vi "OP600ZP_SCANequipements.vi"(8 "Errin":errorcluster caption="errin", 10 "Chaîne":string="Log et conf\\Config.ini", 11 "pathin":path=path "D:/CODE/02 SLIM ZEN") -> (0 "errout":errorcluster={"status"=TRUE, "code"=0, "source"="PCAN_CHANNEL ILLEGAL"}, 1 "KO?":bool=TRUE, 2 "ST5520":refnum<visa-resource-name>, 3 "VISA OUT":T1, 4 "BT3564":refnum<visa-resource-name>, 6 "ALIM":refnum<visa-resource-name>)   [LabVIEW 2020]
doc: "Ce vi il détecte la presence des équipements"
uses:
  VG/VG_BT3564.vi
  VG/VG_ALIM.vi
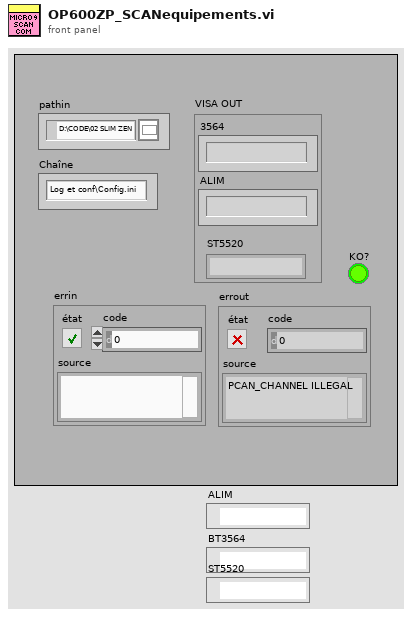
[diagram p1: front panel]
types:
  T1 = cluster{"3564":string, "ALIM":string, "ST5520":string}
  T2 = cluster{"3564":string, "ST5520":string, "ALIM":string}
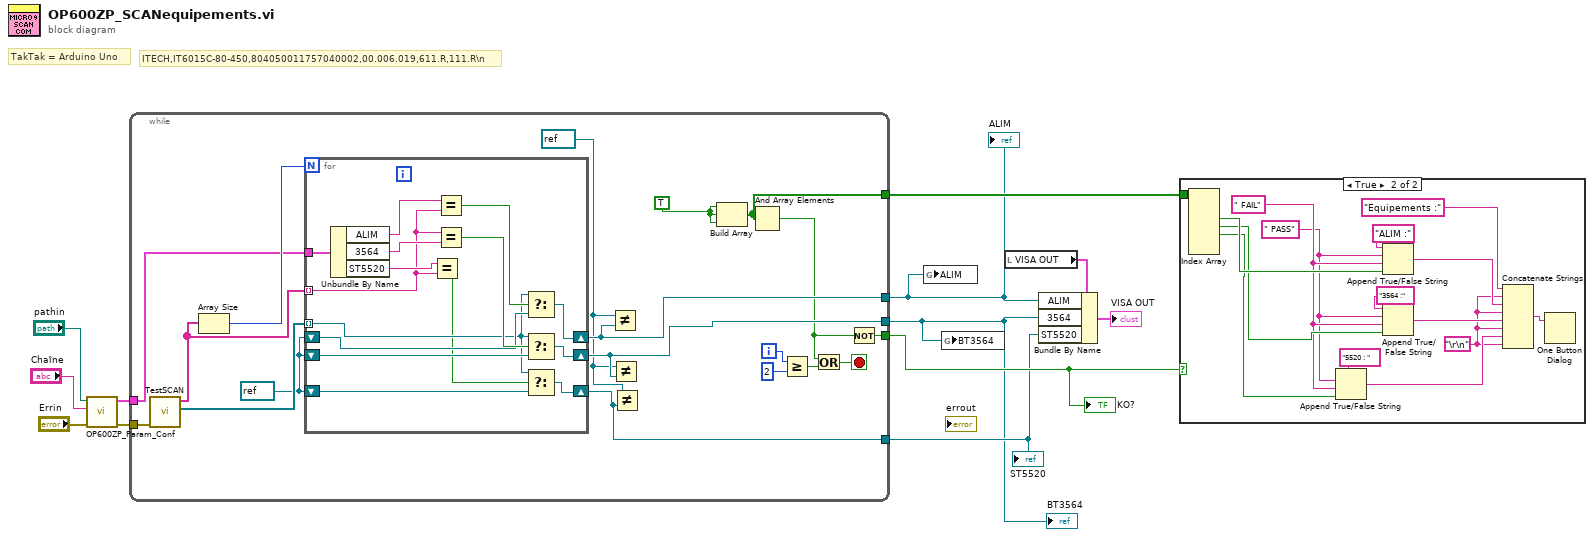
[diagram p0: block diagram]
diagram:
  # "TakTak = Arduino Uno"
  # "ITECH,IT6015C-80-450,804050011757040002,00.006.019,611.R,111.R\\n"
  n1 = call "OP600ZP_Param_Conf.vi"("errin"="Errin", "Chaîne"="Chaîne", "pathin"="pathin") -> ("errout"=w9:errorcluster, "VISA OUT"=w8:T2)  [unwired: 7 in]
  n2 = while {
    tunnel: [w20] -> w2
    tunnel: [w19] -> w1
    tunnel: w9 -> [w29]
    tunnel: [w24] -> w12
    tunnel: w8 -> [w21]
    tunnel: [w17] -> w11
    tunnel: [w14] -> w3
    i -> [w23]
    stop <- w26 stop-if-true
    w13 = TRUE ("élément")
    w15 = refnum<visa-resource-name> refnum ("x")
    w16 = refnum<visa-resource-name> refnum ("VISA resource name out")
    n3 = call <userlib>:"TestSCAN.vi"("errin"=w29) -> ("Tableau 2"=w27:refnum<visa-resource-name>[], "Tableau"=w28:string[])  [unwired: 8 in, 1 out]
    n4 = Array Size(array=w28) -> (size(s)=w30:i32)
    n5 = for {
      N: w30 -> [_]
      shift-right: [w43] -> w20
      shift-left: w16 -> [w41]
      shift-right: [w42] -> w19
      shift-left: w16 -> [w40]
      tunnel: w28 -> [w32] mode=indexing
      tunnel: w21 -> [w39]
      shift-right: [w35] -> w14
      shift-left: w16 -> [w36]
      tunnel: w27 -> [w34] mode=indexing
      n6 = Unbundle By Name(w39) -> ("ALIM"=w38:string, "3564"=w37:string, "ST5520"=w33:string)
      n7 = Equal?(x=w33, y=w32) -> (x = y?=w31:bool)
      n8 = Equal?(x=w38, y=w32) -> (x = y?=w44:bool)
      n9 = Equal?(x=w32, y=w37) -> (x = y?=w45:bool)
      n10 = Select(t=w34, s=w44, f=w41) -> (s? t:f=w43:refnum<visa-resource-name>)
      n11 = Select(t=w34, s=w45, f=w40) -> (s? t:f=w42:refnum<visa-resource-name>)
      n12 = Select(t=w34, s=w31, f=w36) -> (s? t:f=w35:refnum<visa-resource-name>)
    }
    n13 = Not Equal?(x=w15, y=w20) -> ()  [unwired: 1 out]
    n14 = Not Equal?(x=w15, y=w19) -> ()  [unwired: 1 out]
    n15 = Not Equal?(x=w15, y=w14) -> ()  [unwired: 1 out]
    n16 = Build Array(w13, w13, w13) -> (w17:bool[])
    n17 = And Array Elements(Boolean array=w17) -> (logical AND=w18:bool)
    n18 = Greater Or Equal?(x=w23, y=2) -> (x >= y?=w25:bool)
    n19 = Or(x=w18, y=w25) -> (x .or. y?=w26:bool)
    n20 = Not(x=w18) -> (.not. x?=w24:bool)
  }
  "KO?" <- w12
  "ALIM" <- w2
  "BT3564" <- w1
  "ST5520" <- w3
  n21 = global write "VG_ALIM.vi" "ALIM"(w2) -> ()
  n22 = global write "VG_BT3564.vi" "BT3564"(w1) -> ()
  n23 = local read "VISA OUT"() -> (w4:T1)
  n24 = Bundle By Name(cluster=w4, "ALIM"=w2, "3564"=w1, "ST5520"=w3) -> (→"VISA OUT":T1)
  n25 = case shown="True" w12 {
    tunnel: w11 -> [_ w51]
    frame False {
    }
    frame True {
      w52 = "\r\n"
      w46 = " PASS" ("chaîne faux")
      w47 = " FAIL" ("chaîne faux")
      n26 = Index Array(array=w51) -> (element #2=w50:bool, element #3=w49:bool, element #4=w48:bool)  [unwired: 6 in, 3 out]
      n27 = Append True/False String(1:w48, 2:w47, 3:w46, 4:"5520 : " ("chaîne (\"\")")) -> (0:w54:string)
      n28 = Append True/False String(1:w50, 2:w47, 3:w46, 4:"ALIM :" ("chaîne (\"\")")) -> (0:w56:string)
      n29 = Append True/False String(1:w49, 2:w47, 3:w46, 4:"3564 :" ("chaîne (\"\")")) -> (0:w55:string)
      n30 = Concatenate Strings("Equipements :" ("chaîne"), w52, w56, w52, w55, w52, w54, w52) -> (w53:string)
      n31 = One Button Dialog(message=w53) -> ()  [unwired: 1 in, 1 out]
    }
  }
